vi "FillMsgArray.vi"(1 "input array":cluster{i32, "Value":string, i32}[](array[cluster])) -> (0 "output array":cluster{i32, "Value":string, i32}[](array[cluster]))   [LabVIEW 2010]
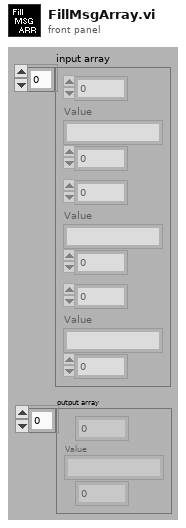
[diagram p1: front panel]
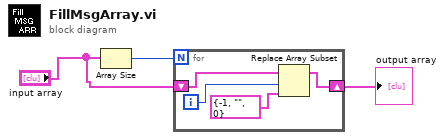
[diagram p0: block diagram]
diagram:
  n1 = Array Size(array="input array") -> (size(s)=w3:i32)
  n2 = for {
    N: w3 -> [_]
    shift-right: [w4] -> w1
    shift-left: "input array" -> [w7]
    i -> [w6]
    n3 = Replace Array Subset(array=w7, new element=cluster{i32, "Value":string, i32} {-1, "Value"="", 0} ("element"), index=w6) -> (w4:cluster{i32, "Value":string, i32}[])
  }
  "output array" <- w1
